vi "Configure Internal Trigger Rate.vi"(0 "VISA resource name":refnum<visa-resource-name>, 5 "Internal Trigger Rate (1 MHz)":dbl=1000000.0 min=0.0 max=10000000.0, 11 "error in (no error)":errorcluster) -> (4 "VISA resource name out":refnum<visa-resource-name>, 15 "error out":errorcluster)   [LabVIEW 2018, in "DG645.lvlib" / "DG645.lvclass"]
doc: "Sets the frequency of the internal trigger to <B>Internal Trigger Rate </B>. \n\n<B>Notes:</B>\nnone"
uses:
  DG645.lvclass
  <instrlib>/Stanford Research DG645/Stanford Research DG645.lvlib
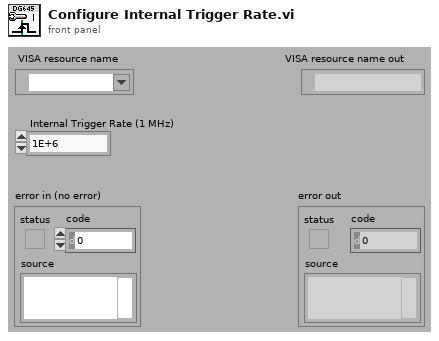
[diagram p1: front panel]
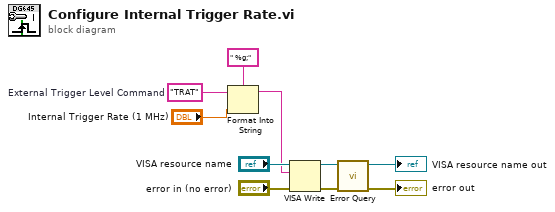
[diagram p0: block diagram]
diagram:
  w4 = "TRAT"  # External Trigger Level Command
  n1 = Format Into String(format string=" %g;" ("Source Command"), initial string=w4, "Internal Trigger Rate (1 MHz)") -> (resulting string=w1:string)  [unwired: 1 in, 1 out]
  n2 = VISA Write(VISA resource name="VISA resource name", write buffer=w1, error in (no error)="error in (no error)") -> (VISA resource name out=w6:refnum<visa-resource-name>, error out=w5:errorcluster)  [unwired: 1 out]
  n3 = call <instrlib>:"Error Query.vi"("error in (no error)"=w5, "VISA resource name"=w6) -> ("error out"=→"error out":errorcluster, "VISA resource name out"=→"VISA resource name out":refnum<visa-resource-name>)  [unwired: 6 in, 2 out]
